vi "Software Update HCC Delete Old Files.vi"(8 "Error In":errorcluster, 9 "folder names":string[](array[string]), 10 "filenames":string[](array[string]), 11 "Path Build List Sub":path) -> (0 "Error Out":errorcluster)   [LabVIEW 2016]
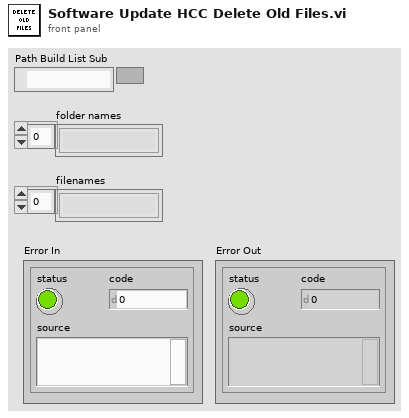
[diagram p1: front panel]
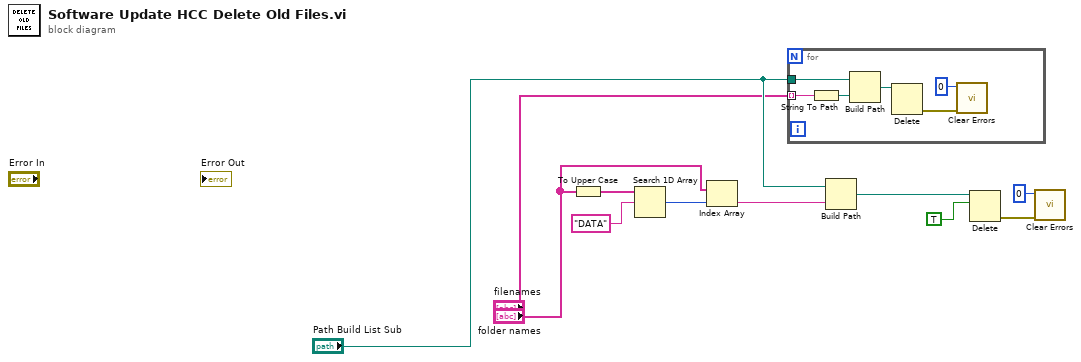
[diagram p0: block diagram]
diagram:
  n1 = To Upper Case(1:"folder names") -> (0:w2:string[])
  n2 = Search 1D Array(1D array=w2, element="DATA") -> (index of element=w4:i32)  [unwired: 1 in]
  n3 = Index Array(array="folder names", index=w4) -> (element=w7:string)
  n4 = for {
    tunnel: "filenames" -> [w17] mode=indexing
    tunnel: "Path Build List Sub" -> [w12]
    n5 = String To Path(string=w17) -> (path=w16:path)
    n6 = Build Path(base path=w12, name or relative path=w16) -> (appended path=w15:path)
    n7 = Delete(path (use dialog)=w15) -> (error out=w14:errorcluster)  [unwired: 4 in, 2 out]
    n8 = call <vilib>:"Clear Errors.vi"("error in (no error)"=w14, "specific error code to clear (0: all)"=0) -> ()  [unwired: 4 in, 2 out]
  }
  n9 = Build Path(base path="Path Build List Sub", name or relative path=w7) -> (appended path=w10:path)
  n10 = Delete(path (use dialog)=w10, entire hierarchy (F)=TRUE) -> (error out=w9:errorcluster)  [unwired: 3 in, 2 out]
  n11 = call <vilib>:"Clear Errors.vi"("error in (no error)"=w9, "specific error code to clear (0: all)"=0) -> ()  [unwired: 4 in, 2 out]
